vi "SetCursor.vi"(0 "reference in":refnum<class "LcPictureBox.lvclass">, 2 "CursorType":T1, 5 "error in (no error)":errorcluster) -> (14 "reference out":refnum<class "LcPictureBox.lvclass">, 19 "error out":errorcluster)   [LabVIEW 2020, in "LcPictureBox.lvclass"]
uses:
  LcPictureBox.lvclass
  System.Windows.Forms
  CursorType.ctl
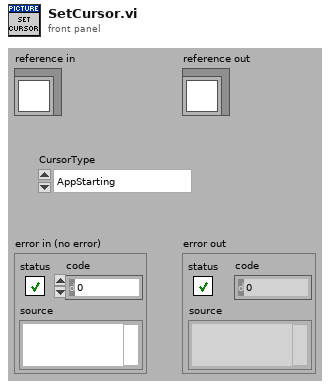
[diagram p1: front panel]
types:
  T1 = typedef "LcPictureBox.lvclass/CursorType.ctl" = enum16{"AppStarting", "Arrow", "Cross", "Default", "Hand", "Help", "HSplit", "IBeam", "No", "NoMove2D", "NoMoveHoriz", "NoMoveVert", "PanEast", "PanNE", "PanNorth", "PanNW", "PanSE", "PanSouth", "PanSW", "PanWest", "SizeAll", "SizeNESW", "SizeNS", "SizeNWSE", "SizeWE", "UpArrow", "VSplit", "WaitCursor"}
  T2 = typedef "LcPictureBox.lvclass/ObjectAttributes.ctl" = cluster{"PictureBox":refnum<k24>, "ImageSize":cluster{"Width":i32, "Height":i32}, "PenMemory":map{cluster{"Alpha(100%)":dbl, "Color(Black)":u32, "Pen(Width=1, Solid)":T3}, refnum<k24>}, "GraphicsRef":refnum<k24>, "BrushMemory":map{cluster{"Alpha(100%)":dbl, "Color(Black)":u32}, refnum<k24>}, "Images":refnum<k24>[], "ImageIndex":i32, "BgColor(None)":u32, "LoadedImages":map{string, cluster{"ImageOut":refnum<k24>, "ImageSize":cluster{"Width":i32, "Height":i32}}}, "ColorsMemory":map{cluster{"Alpha(100%)":dbl, "Color(Black)":u32}, refnum<k24>}, "CacheSize":i32, "PictureBoxActiveXReference":refnum<vi>, "Scale":sgl, "Offset":cluster{"x":sgl, "y":sgl}, "zoom_center":cluster{"X":i32, "Y":i32}, "ImagesCreated":refnum<k24>[]}
  T3 = typedef "LcPictureBox.lvclass/Pen.ctl" = cluster{"Width":u16, "Style":enum32{"Solid", "Dash", "Dot", "DashDot", "DashDotDot"}}
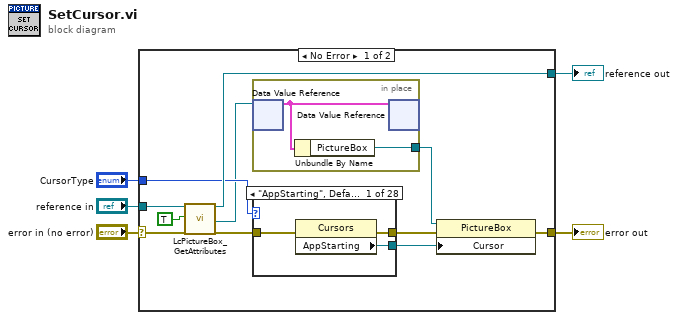
[diagram p0: block diagram]
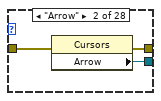
[diagram p2: hidden frame]
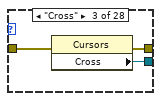
[diagram p3: hidden frame]
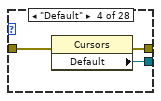
[diagram p4: hidden frame]
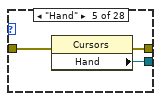
[diagram p5: hidden frame]
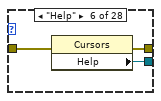
[diagram p6: hidden frame]
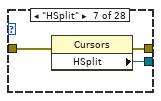
[diagram p7: hidden frame]
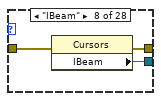
[diagram p8: hidden frame]
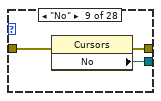
[diagram p9: hidden frame]
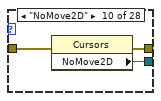
[diagram p10: hidden frame]
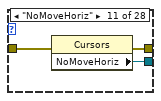
[diagram p11: hidden frame]
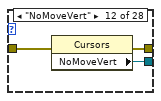
[diagram p12: hidden frame]
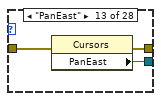
[diagram p13: hidden frame]
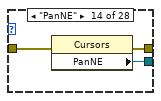
[diagram p14: hidden frame]
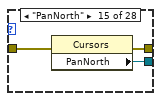
[diagram p15: hidden frame]
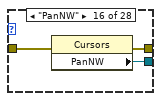
[diagram p16: hidden frame]
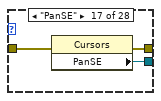
[diagram p17: hidden frame]
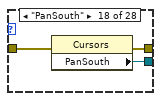
[diagram p18: hidden frame]
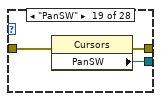
[diagram p19: hidden frame]
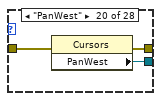
[diagram p20: hidden frame]
diagram:
  n1 = case shown="No Error" "error in (no error)" {
    selector: "error in (no error)" -> [w16 w104]
    tunnel: [w9 w104] -> w4
    tunnel: [w14 w103] -> w2
    tunnel: "reference in" -> [w15 w103]
    tunnel: "CursorType" -> [w13 _]
    frame No Error {
      n2 = call "LcPictureBox_GetAttributes.vi"("reference in"=w15, "OnlyGetDvrReference(False)"=TRUE, "error in (no error)"=w16) -> ("reference out"=w14:refnum<class "LcPictureBox.lvclass">, "DataRef"=w7:refnum<data-value>, "error out"=w10:errorcluster)  [unwired: 13 in, 1 out]
      n3 = in-place {
        in-place-border: [w18] -> w6
        n4 = in-place-dvr #1(w7) -> (w17:T2)  [unwired: 1 out]
        n5 = Unbundle By Name(w17) -> ("PictureBox"=w18:refnum<k24>)
        n6 = in-place-dvr #1(w17) -> ()  [unwired: 2 out]
      }
      n7 = case shown="\"AppStarting\", Default" w13 {
        tunnel: [w21 w24 w27 w30 w33 w36 w39 w42 w45 w48 w51 w54 w57 w60 w63 w66 w69 w72 w75 w78 w81 w84 w87 w90 w93 w96 w99 w102] -> w12
        tunnel: [w20 w23 w26 w29 w32 w35 w38 w41 w44 w47 w50 w53 w56 w59 w62 w65 w68 w71 w74 w77 w80 w83 w86 w89 w92 w95 w98 w101] -> w11
        tunnel: w10 -> [w19 w22 w25 w28 w31 w34 w37 w40 w43 w46 w49 w52 w55 w58 w61 w64 w67 w70 w73 w76 w79 w82 w85 w88 w91 w94 w97 w100]
        frame "AppStarting", Default {
          n8 = property class="Cursors"(error in=w19) -> (error out=w20:errorcluster, "AppStarting"=w21:refnum<k24>)  [unwired: 1 in, 1 out]
        }
        frame "Arrow" {
          n9 = property class="Cursors"(error in=w22) -> (error out=w23:errorcluster, "Arrow"=w24:refnum<k24>)  [unwired: 1 in, 1 out]
        }
        frame "Cross" {
          n10 = property class="Cursors"(error in=w25) -> (error out=w26:errorcluster, "Cross"=w27:refnum<k24>)  [unwired: 1 in, 1 out]
        }
        frame "Default" {
          n11 = property class="Cursors"(error in=w28) -> (error out=w29:errorcluster, "Default"=w30:refnum<k24>)  [unwired: 1 in, 1 out]
        }
        frame "Hand" {
          n12 = property class="Cursors"(error in=w31) -> (error out=w32:errorcluster, "Hand"=w33:refnum<k24>)  [unwired: 1 in, 1 out]
        }
        frame "Help" {
          n13 = property class="Cursors"(error in=w34) -> (error out=w35:errorcluster, "Help"=w36:refnum<k24>)  [unwired: 1 in, 1 out]
        }
        frame "HSplit" {
          n14 = property class="Cursors"(error in=w37) -> (error out=w38:errorcluster, "HSplit"=w39:refnum<k24>)  [unwired: 1 in, 1 out]
        }
        frame "IBeam" {
          n15 = property class="Cursors"(error in=w40) -> (error out=w41:errorcluster, "IBeam"=w42:refnum<k24>)  [unwired: 1 in, 1 out]
        }
        frame "No" {
          n16 = property class="Cursors"(error in=w43) -> (error out=w44:errorcluster, "No"=w45:refnum<k24>)  [unwired: 1 in, 1 out]
        }
        frame "NoMove2D" {
          n17 = property class="Cursors"(error in=w46) -> (error out=w47:errorcluster, "NoMove2D"=w48:refnum<k24>)  [unwired: 1 in, 1 out]
        }
        frame "NoMoveHoriz" {
          n18 = property class="Cursors"(error in=w49) -> (error out=w50:errorcluster, "NoMoveHoriz"=w51:refnum<k24>)  [unwired: 1 in, 1 out]
        }
        frame "NoMoveVert" {
          n19 = property class="Cursors"(error in=w52) -> (error out=w53:errorcluster, "NoMoveVert"=w54:refnum<k24>)  [unwired: 1 in, 1 out]
        }
        frame "PanEast" {
          n20 = property class="Cursors"(error in=w55) -> (error out=w56:errorcluster, "PanEast"=w57:refnum<k24>)  [unwired: 1 in, 1 out]
        }
        frame "PanNE" {
          n21 = property class="Cursors"(error in=w58) -> (error out=w59:errorcluster, "PanNE"=w60:refnum<k24>)  [unwired: 1 in, 1 out]
        }
        frame "PanNorth" {
          n22 = property class="Cursors"(error in=w61) -> (error out=w62:errorcluster, "PanNorth"=w63:refnum<k24>)  [unwired: 1 in, 1 out]
        }
        frame "PanNW" {
          n23 = property class="Cursors"(error in=w64) -> (error out=w65:errorcluster, "PanNW"=w66:refnum<k24>)  [unwired: 1 in, 1 out]
        }
        frame "PanSE" {
          n24 = property class="Cursors"(error in=w67) -> (error out=w68:errorcluster, "PanSE"=w69:refnum<k24>)  [unwired: 1 in, 1 out]
        }
        frame "PanSouth" {
          n25 = property class="Cursors"(error in=w70) -> (error out=w71:errorcluster, "PanSouth"=w72:refnum<k24>)  [unwired: 1 in, 1 out]
        }
        frame "PanSW" {
          n26 = property class="Cursors"(error in=w73) -> (error out=w74:errorcluster, "PanSW"=w75:refnum<k24>)  [unwired: 1 in, 1 out]
        }
        frame "PanWest" {
          n27 = property class="Cursors"(error in=w76) -> (error out=w77:errorcluster, "PanWest"=w78:refnum<k24>)  [unwired: 1 in, 1 out]
        }
        frame "SizeAll" {
          n28 = property class="Cursors"(error in=w79) -> (error out=w80:errorcluster, "SizeAll"=w81:refnum<k24>)  [unwired: 1 in, 1 out]
        }
        frame "SizeNESW" {
          n29 = property class="Cursors"(error in=w82) -> (error out=w83:errorcluster, "SizeNESW"=w84:refnum<k24>)  [unwired: 1 in, 1 out]
        }
        frame "SizeNS" {
          n30 = property class="Cursors"(error in=w85) -> (error out=w86:errorcluster, "SizeNS"=w87:refnum<k24>)  [unwired: 1 in, 1 out]
        }
        frame "SizeNWSE" {
          n31 = property class="Cursors"(error in=w88) -> (error out=w89:errorcluster, "SizeNWSE"=w90:refnum<k24>)  [unwired: 1 in, 1 out]
        }
        frame "SizeWE" {
          n32 = property class="Cursors"(error in=w91) -> (error out=w92:errorcluster, "SizeWE"=w93:refnum<k24>)  [unwired: 1 in, 1 out]
        }
        frame "UpArrow" {
          n33 = property class="Cursors"(error in=w94) -> (error out=w95:errorcluster, "UpArrow"=w96:refnum<k24>)  [unwired: 1 in, 1 out]
        }
        frame "VSplit" {
          n34 = property class="Cursors"(error in=w97) -> (error out=w98:errorcluster, "VSplit"=w99:refnum<k24>)  [unwired: 1 in, 1 out]
        }
        frame "WaitCursor" {
          n35 = property class="Cursors"(error in=w100) -> (error out=w101:errorcluster, "WaitCursor"=w102:refnum<k24>)  [unwired: 1 in, 1 out]
        }
      }
      n36 = property class="PictureBox"(reference=w6, error in=w11, "Cursor"=w12) -> (error out=w9:errorcluster)  [unwired: 1 out]
    }
    frame Error {
    }
  }
  "error out" <- w4
  "reference out" <- w2
